vi "Close.vi"(6 "CloseHeaders":bool, 8 "error in (no error)":errorcluster, 11 "HttpResponseMessage in":refnum<class "HttpResponseMessage.lvclass">) -> (0 "error out":errorcluster)   [LabVIEW 2018, in "HttpClient_NET.lvlib" / "HttpResponseMessage.lvclass"]
doc: "<b> </b> <b> </b>\nHttpClient_NET\nJustin Young - Viviota\nCopyright (c) 2021\nLicense: BSD"
uses:
  HttpResponseMessage.lvclass
  HttpResponseMessage.lvclass/HttpResponseMessage.ctl
  Accessors/Read NET_HttpResponseTask.vi
  Accessors/Read NET_CancellationSource.vi
  Accessors/Read NET_HttpReponseMessage.vi
  Accessors/Read HttpContent.vi
  Accessors/Read HttpHeaders_Response.vi
  Accessors/Read HttpRequestMessage.vi
  HttpHeaders_response/HttpHeaders_Response.lvclass
  C:/Viviota/Projects/R&D/__OpenSource/VIV_HTTP_REST_NET/HTTPHeaders_NET/HttpHeaders_NET.lvclass
  System.Net.Http
  HttpContent/HttpContent.lvclass
  HttpRequestMessage/HttpRequestMessage.lvclass
  HTTPHeaders_NET/HttpHeaders_NET.lvclass
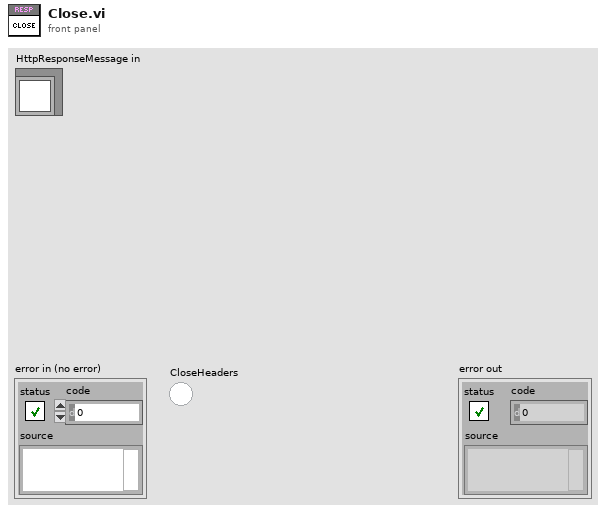
[diagram p1: front panel]
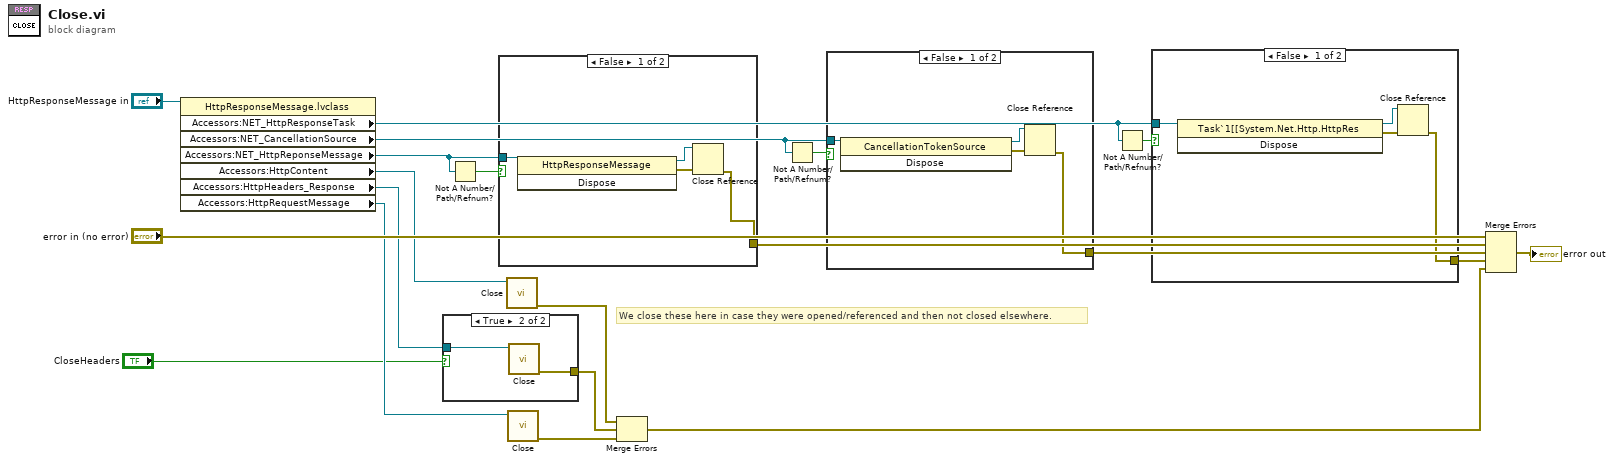
[diagram p0: block diagram]
diagram:
  # "We close these here in case they were opened/referenced and then not closed elsewhere."
  n1 = property class="HttpResponseMessage.lvclass"(reference="HttpResponseMessage in") -> ("Accessors:NET_HttpResponseTask"=w12:refnum<k24>, "Accessors:NET_CancellationSource"=w13:refnum<k24>, "Accessors:NET_HttpReponseMessage"=w14:refnum<k24>, "Accessors:HttpContent"=w6:refnum<class "HttpContent.lvclass">, "Accessors:HttpHeaders_Response"=w7:refnum<class "HttpHeaders_Response.lvclass">, "Accessors:HttpRequestMessage"=w8:refnum<class "HttpRequestMessage.lvclass">)  [unwired: 1 in, 2 out]
  n2 = case shown="True" "CloseHeaders" {
    tunnel: w7 -> [_ w22]
    tunnel: [_ w21] -> w4
    frame False {
    }
    frame True {
      n3 = call "Close.vi"("HTTPHeaders_NET in"=w22) -> ("error out"=w21:errorcluster)  [unwired: 10 in]
    }
  }
  n4 = Not A Number/Path/Refnum?(number/path/refnum=w14) -> (NaN/Path/Refnum?=w11:bool)
  n5 = case shown="False" w11 {
    tunnel: [w24 _] -> w17
    tunnel: w14 -> [w23 _]
    frame False {
      n6 = invoke class="HttpResponseMessage" method="Dispose"(reference=w23) -> (reference out=w25:refnum<k24>, error out=w26:errorcluster)  [unwired: 2 in, 1 out]
      n7 = Close Reference(reference=w25, error in (no error)=w26) -> (error out=w24:errorcluster)
    }
    frame True {
    }
  }
  n8 = call "Close.vi"("HttpContent in"=w6) -> ("error out"=w3:errorcluster)  [unwired: 10 in]
  n9 = call "Close.vi"("RequestMessage"=w8) -> ("Error Out"=w5:errorcluster)  [unwired: 10 in]
  n10 = Merge Errors(w3, w4, w5) -> (w2:errorcluster)
  n11 = Not A Number/Path/Refnum?(number/path/refnum=w13) -> (NaN/Path/Refnum?=w10:bool)
  n12 = case shown="False" w10 {
    tunnel: [w28 _] -> w16
    tunnel: w13 -> [w27 _]
    frame False {
      n13 = invoke class="CancellationTokenSource" method="Dispose"(reference=w27) -> (reference out=w29:refnum<k24>, error out=w30:errorcluster)  [unwired: 2 in, 1 out]
      n14 = Close Reference(reference=w29, error in (no error)=w30) -> (error out=w28:errorcluster)
    }
    frame True {
    }
  }
  n15 = Not A Number/Path/Refnum?(number/path/refnum=w12) -> (NaN/Path/Refnum?=w9:bool)
  n16 = case shown="False" w9 {
    tunnel: [w32 _] -> w15
    tunnel: w12 -> [w31 _]
    frame False {
      n17 = invoke class="Task`1[[System.Net.Http.HttpRes" method="Dispose"(reference=w31) -> (reference out=w33:refnum<k24>, error out=w34:errorcluster)  [unwired: 2 in, 1 out]
      n18 = Close Reference(reference=w33, error in (no error)=w34) -> (error out=w32:errorcluster)
    }
    frame True {
    }
  }
  n19 = Merge Errors("error in (no error)", w17, w16, w15, w2) -> (→"error out":errorcluster)
